vi "Check RPM.vi"(8 "% Difference":dbl, 10 "Motor Input":dbl, 11 "RPM":dbl) -> (3 "RPM Drop":bool)   [LabVIEW 2013]
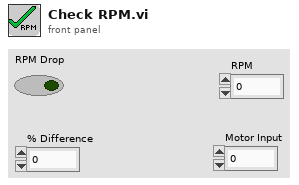
[diagram p1: front panel]
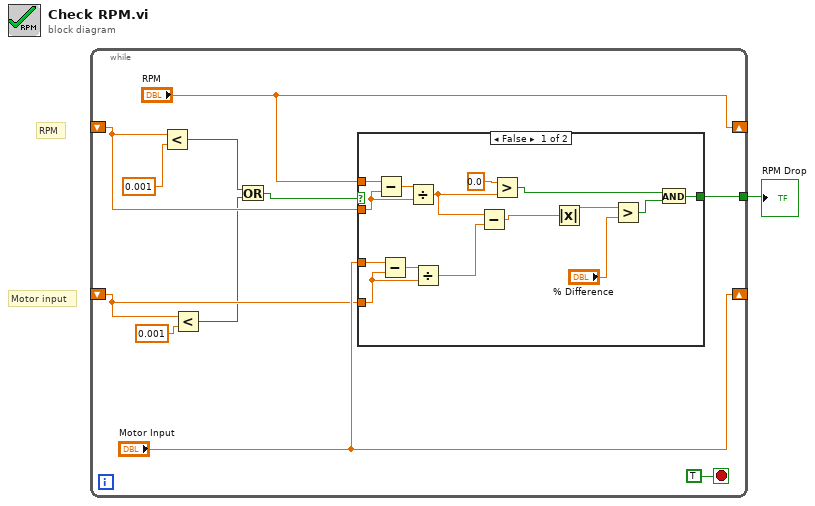
[diagram p0: block diagram]
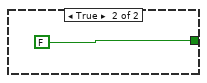
[diagram p2: hidden frame]
diagram:
  # "Motor input"
  # "RPM"
  n1 = while {
    shift-right: ["RPM"] -> _
    shift-left: _ -> [w5]
    shift-right: ["Motor Input"] -> _
    shift-left: _ -> [w7]
    tunnel: [w9] -> w1
    stop <- TRUE stop-if-true
    n2 = Less?(x=w5, y=0.001) -> (x < y?=w4:bool)
    n3 = Less?(x=w7, y=0.001) -> (x < y?=w3:bool)
    n4 = Or(x=w4, y=w3) -> (x .or. y?=w2:bool)
    n5 = case shown="False" w2 {
      tunnel: [w15 FALSE] -> w9
      tunnel: "Motor Input" -> [w24 _]
      tunnel: w7 -> [w22 _]
      tunnel: "RPM" -> [w27 _]
      tunnel: w5 -> [w25 _]
      frame False {
        n6 = Subtract(x=w27, y=w25) -> (x-y=w26:dbl)
        n7 = Subtract(x=w24, y=w22) -> (x-y=w23:dbl)
        n8 = Divide(x=w26, y=w25) -> (x/y=w16:dbl)
        n9 = Divide(x=w23, y=w22) -> (x/y=w20:dbl)
        n10 = Subtract(x=w16, y=w20) -> (x-y=w19:dbl)
        n11 = Greater?(x=0.0 ("y"), y=w16) -> (0:w13:bool)
        n12 = Absolute Value(x=w19) -> (abs(x)=w21:dbl)
        n13 = Greater?(x=w21, y="% Difference") -> (0:w14:bool)
        n14 = And(x=w13, y=w14) -> (x .and. y?=w15:bool)
      }
      frame True {
      }
    }
  }
  "RPM Drop" <- w1
